vi "append data log.vi"(0 "file refnum in":refnum<file>, 7 "Power":dbl=1.0 format="%.2f", 9 "Temp":dbl format="%.2f", 11 "Control Parameters":T1={"Setpoint"=50.0, "Control bandwidth"=4.0, "Settle bandwidth"=1.0, "Integral time"=30.0, "Int\non"=TRUE, "Derivative time"=0.5, "Der\non"=TRUE, "Settle time"=60.0} {"Settle time" format="%.2f"; "Derivative time" format="%.2f"; "Integral time" format="%.2f"; "Settle bandwidth" format="%.2f"; "Control bandwidth" format="%.2f"; "Setpoint" format="%.2f"}) -> ()   [LabVIEW 2016]
doc: "This vi adds an entry to the data log using the current experiment data\n\nPaul K Dixon\nPhysics 350\nPaul K Dixon"
uses:
  typedefs/control parameters.ctl
  <vilib>/Utility/file.llb/Write Delimited Spreadsheet (DBL).vi
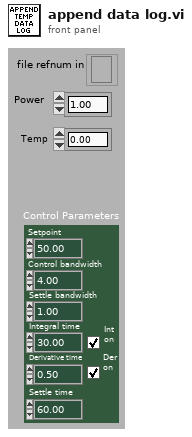
[diagram p1: front panel]
types:
  T1 = typedef "control parameters.ctl" = cluster{"Setpoint":dbl, "Control bandwidth":dbl, "Settle bandwidth":dbl, "Integral time":dbl, "Int\non":bool, "Derivative time":dbl, "Der\non":bool, "Settle time":dbl}
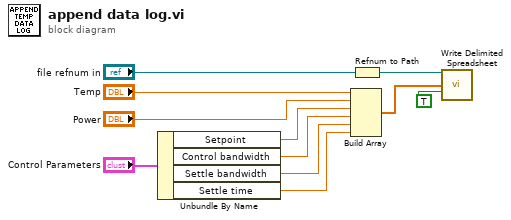
[diagram p0: block diagram]
diagram:
  n1 = Unbundle By Name("Control Parameters") -> ("Setpoint"=w8:dbl, "Control bandwidth"=w7:dbl, "Settle bandwidth"=w6:dbl, "Settle time"=w5:dbl)
  n2 = Build Array("Temp", "Power", w8, w7, w6, w5) -> (w9:dbl[])
  n3 = Refnum to Path(1:"file refnum in") -> (0:w11:path)
  n4 = call-poly <vilib>:"Write Delimited Spreadsheet.vi"("file path (dialog if empty)"=w11, "1D data"=w9, "append to file? (new file:F)"=TRUE) -> ()  [unwired: 11 in, 2 out]
